vi "Check Published Group.vi"(8 "error in (no error)":errorcluster, 11 "Data Processor Module in":refnum<class "Data Processor Module.lvclass">) -> (0 "error out":errorcluster, 3 "Data Processor Module out":refnum<class "Data Processor Module.lvclass">)   [LabVIEW 2020, in "VolatusData.lvlib" / "Data Processor Module.lvclass"]
uses:
  Data Processor Module.lvclass
  lv-vecto/Vecto/Publish Config.ctl
  Data Processor Module.lvclass/Data Processor Module.ctl
  lv-vecto/Vecto/Group/Group.lvclass/Group.ctl
  lv-vecto/Vecto/Group/Group.lvclass
  lv-vecto/Vecto/Group Config/Group Config.lvclass
  lv-vecto/VectoConfig/VectoConfig.lvlib
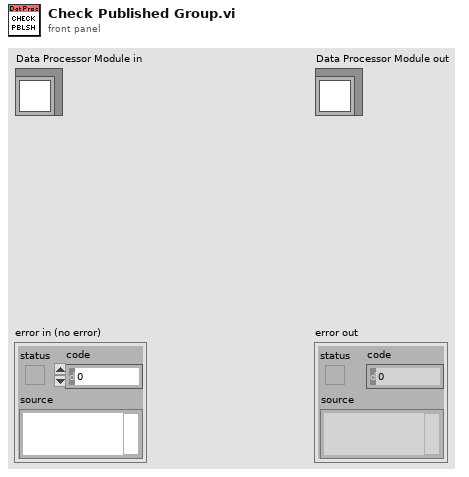
[diagram p1: front panel]
types:
  T1 = typedef "VectoConfig.lvlib/Publish Config.ctl" = cluster{"Address":string, "Port":u16}
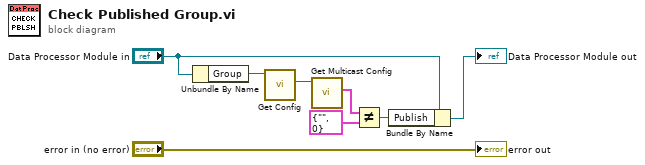
[diagram p0: block diagram]
diagram:
  n1 = Unbundle By Name("Data Processor Module in") -> ("Group"=w7:refnum<class "Group.lvclass">)
  n2 = call "Get Config.vi"("Group in"=w7) -> ("Config"=w6:refnum<class "Group Config.lvclass">)  [unwired: 8 in, 2 out]
  n3 = call "Get Multicast Config.vi"("Group Config in"=w6) -> ("Multicast Config"=w5:T1)  [unwired: 8 in, 2 out]
  n4 = Not Equal?(x=w5, y=T1 {"Address"="", "Port"=0}) -> (x != y?=w3:bool)
  n5 = Bundle By Name(cluster="Data Processor Module in", "Publish"=w3) -> (→"Data Processor Module out":refnum<class "Data Processor Module.lvclass">)
  "error out" <- "error in (no error)"
